vi "sub vi - Read Analog All v8.11.vi"() -> (2 "Analog loop time":dbl, 3 "array GRAPH":dynamicdata[](array[waveform]), 4 "LAB01":T2, 6 "LAB02":T3, 8 "LAB03":T4, 10 "LAB04":T5, 14 "array ERROR":errorcluster[](array[cluster]), 15 "LAB05":T6)   [LabVIEW 2013]
uses:
  program files/Global display 3.vi
  <vilib>/measure/mascope.llb/Amplitude and Levels 1 chan.vi
  <vilib>/addons/Electrical Power/Basic/Measurement/Power (1 Channel).vi
  <vilib>/addons/Electrical Power/Basic/Measurement/RMS (N Channels).vi
  <vilib>/addons/Electrical Power/Basic/NI_EP_Basic.lvlib
  <vilib>/measure/NI_MAPro.lvlib
panel:
  in  "Tab Control":T1(tab)
  out "LAB01-2 (PF)":dbl
  out "LAB01-1 (PF)":dbl
  out "LAB01-2 (V)":dbl
  out "LAB01-2 (A)":dbl
  out "LAB01-1 (V)":dbl
  out "LAB01-1 (A)":dbl
  out "LAB01-2 (GRAPH)":dynamicdata(graph)
  out "LAB01-1 (GRAPH)":dynamicdata(graph)
  out "LAB02-2 (PF)":dbl
  out "LAB02-1 (PF)":dbl
  out "LAB02-2 (V)":dbl
  out "LAB02-2 (A)":dbl
  out "LAB02-1 (V)":dbl
  out "LAB02-1 (A)":dbl
  out "LAB02-2 (GRAPH)":dynamicdata(graph)
  out "LAB02-1 (GRAPH)":dynamicdata(graph)
  out "LAB03-2 (PF)":dbl
  out "LAB03-1 (PF)":dbl
  out "LAB03-2 (V)":dbl
  out "LAB03-2 (A)":dbl
  out "LAB03-1 (V)":dbl
  out "LAB03-1 (A)":dbl
  out "LAB03-2 (GRAPH)":dynamicdata(graph)
  out "LAB03-1 (GRAPH)":dynamicdata(graph)
  out "LAB04-2 (PF)":dbl
  out "LAB04-1 (PF)":dbl
  out "LAB04-2 (V)":dbl
  out "LAB04-2 (A)":dbl
  out "LAB04-1 (V)":dbl
  out "LAB04-1 (A)":dbl
  out "LAB04-1 (GRAPH)":dynamicdata(graph)
  out "LAB04-2 (GRAPH)":dynamicdata(graph)
  out "LAB05-2 (PF)":dbl
  out "LAB05-1 (PF)":dbl
  out "LAB05-2 (V)":dbl
  out "LAB05-2 (A)":dbl
  out "LAB05-1 (V)":dbl
  out "LAB05-1 (A)":dbl
  out "LAB05-1 (GRAPH)":dynamicdata(graph)
  out "LAB05-2 (GRAPH)":dynamicdata(graph)
  out "A1 error":errorcluster
  out "AI2-OFF":dynamicdata(graph)
  out "AI2-ON":dynamicdata(graph)
  out "AI1-OFF":dynamicdata(graph)
  out "AI1-ON":dynamicdata(graph)
  out "AI0-OFF":dynamicdata(graph)
  out "AI0-ON":dynamicdata(graph)
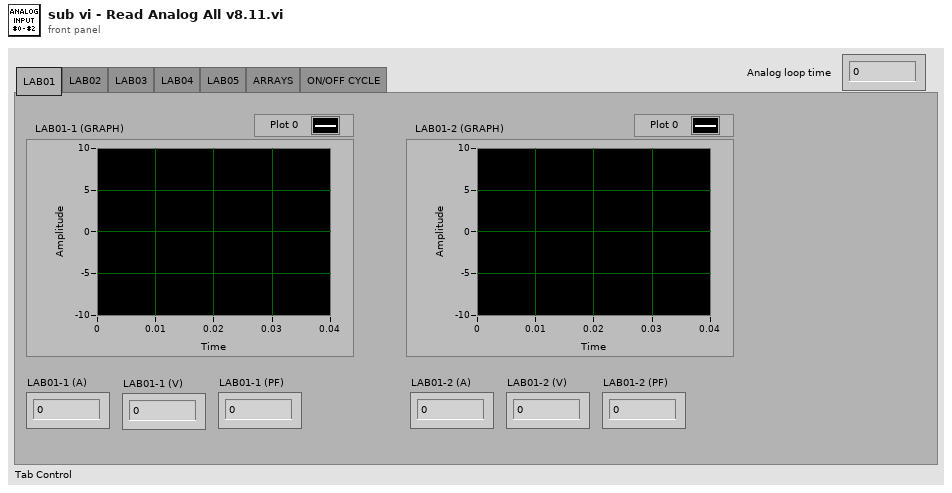
[diagram p1: front panel]
types:
  T1 = enum32{"LAB01", "LAB02", "LAB03", "LAB04", "LAB05", "ARRAYS", "ON/OFF CYCLE"}
  T2 = cluster{"LAB01-1 (A)":dbl, "LAB01-1 (V)":dbl, "LAB01-1 (PF)":dbl, "LAB01-2 (A)":dbl, "LAB01-2 (V)":dbl, "LAB01-2 (PF)":dbl}
  T3 = cluster{"LAB02-1 (A)":dbl, "LAB02-1 (V)":dbl, "LAB02-1 (PF)":dbl, "LAB02-2 (A)":dbl, "LAB02-2 (V)":dbl, "LAB02-2 (PF)":dbl}
  T4 = cluster{"LAB03-1 (A)":dbl, "LAB03-1 (V)":dbl, "LAB03-1 (PF)":dbl, "LAB03-2 (A)":dbl, "LAB03-2 (V)":dbl, "LAB03-2 (PF)":dbl}
  T5 = cluster{"LAB04-1 (A)":dbl, "LAB04-1 (V)":dbl, "LAB04-1 (PF)":dbl, "LAB04-2 (A)":dbl, "LAB04-2 (V)":dbl, "LAB04-2 (PF)":dbl}
  T6 = cluster{"LAB05-1 (A)":dbl, "LAB05-1 (V)":dbl, "LAB05-1 (PF)":dbl, "LAB05-2 (A)":dbl, "LAB05-2 (V)":dbl, "LAB05-2 (PF)":dbl}
  T7 = typedef "NI_EP_Basic.lvlib/basic_Power Value.ctl" = cluster{"active power [W]":dbl, "apparent power [VA]":dbl, "reactive power [VAR]":dbl, "power factor":dbl}
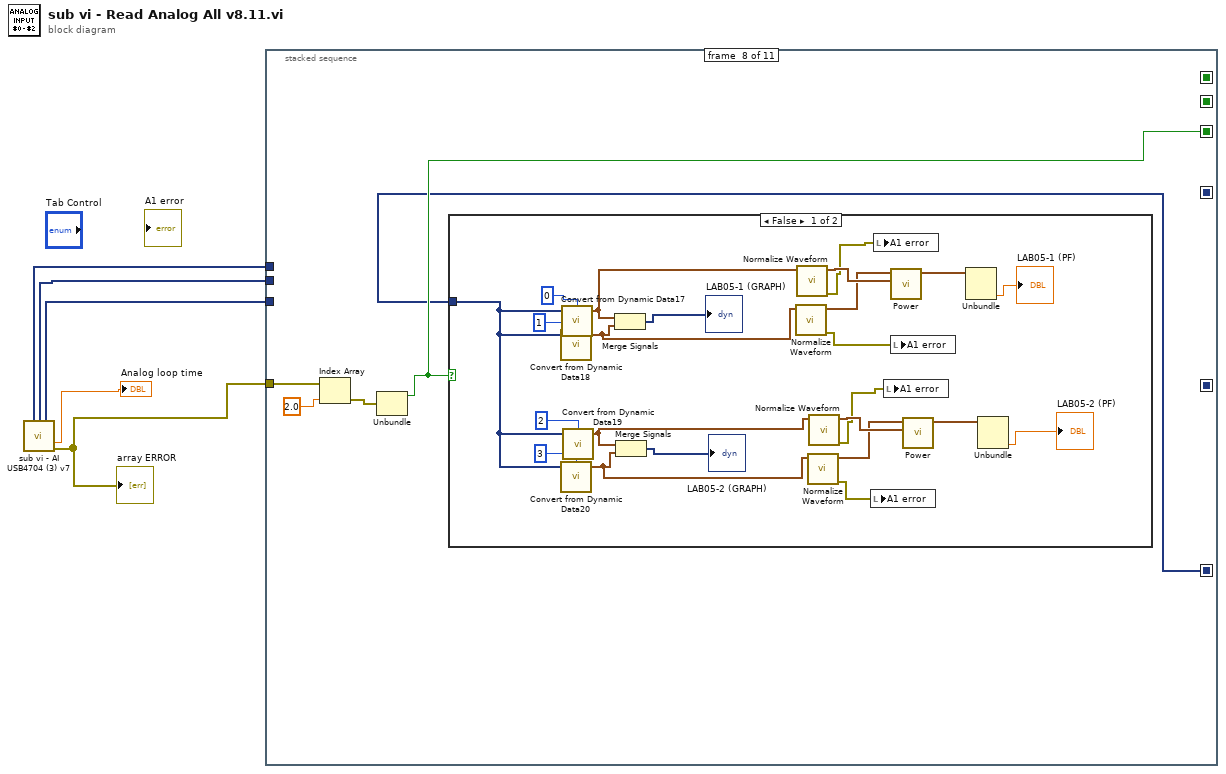
[diagram p0: block diagram]
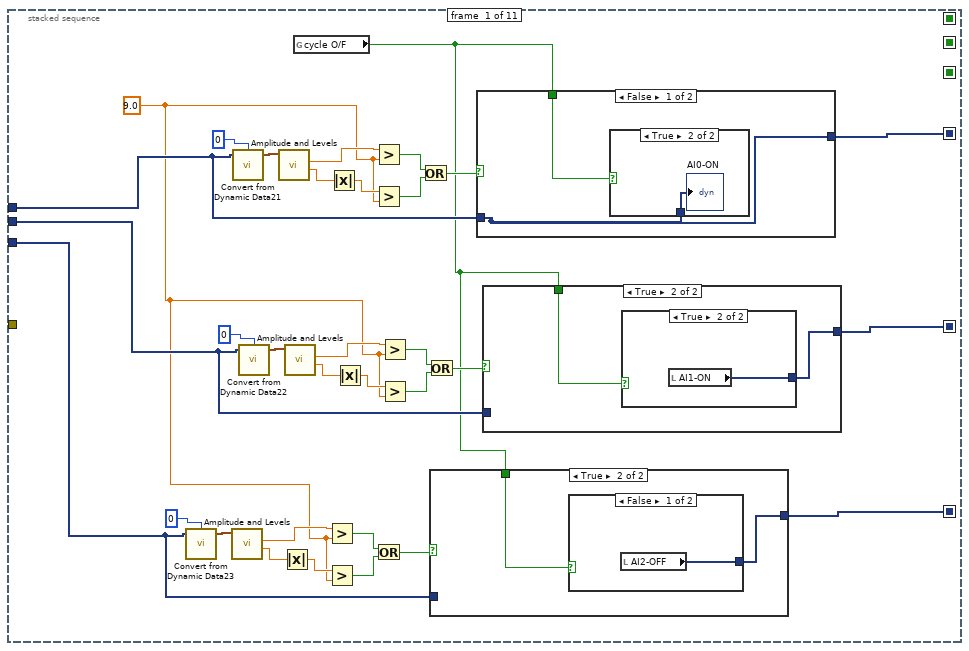
[diagram p2: hidden frame]
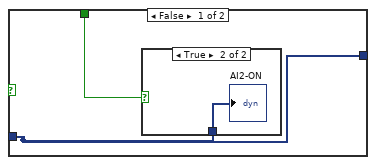
[diagram p3: hidden frame]
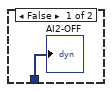
[diagram p4: hidden frame]
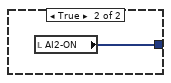
[diagram p5: hidden frame]
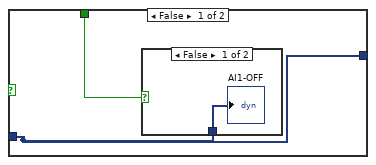
[diagram p6: hidden frame]
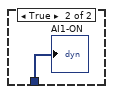
[diagram p7: hidden frame]
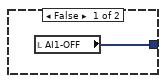
[diagram p8: hidden frame]
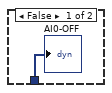
[diagram p9: hidden frame]
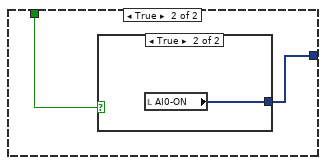
[diagram p10: hidden frame]
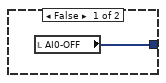
[diagram p11: hidden frame]
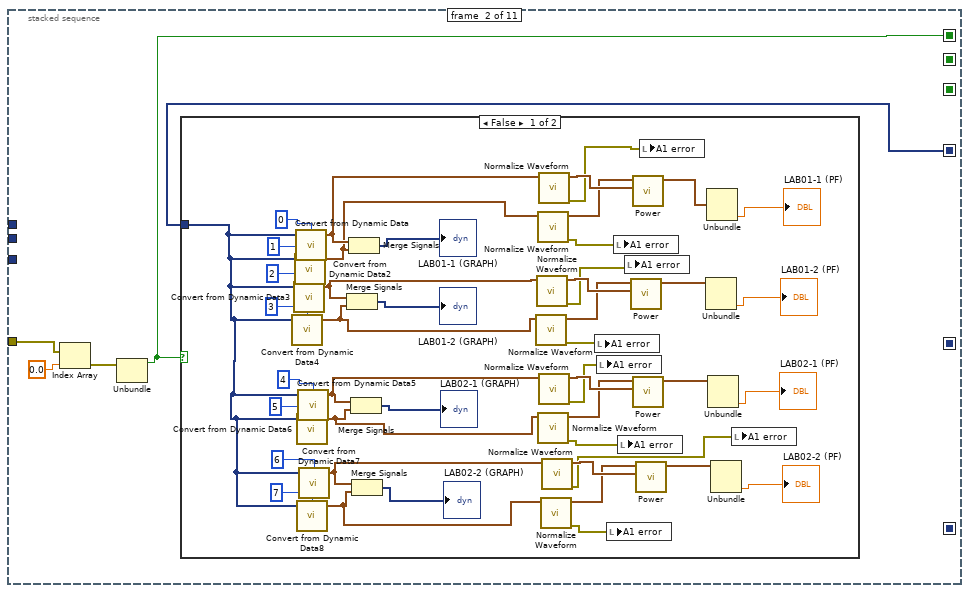
[diagram p12: hidden frame]
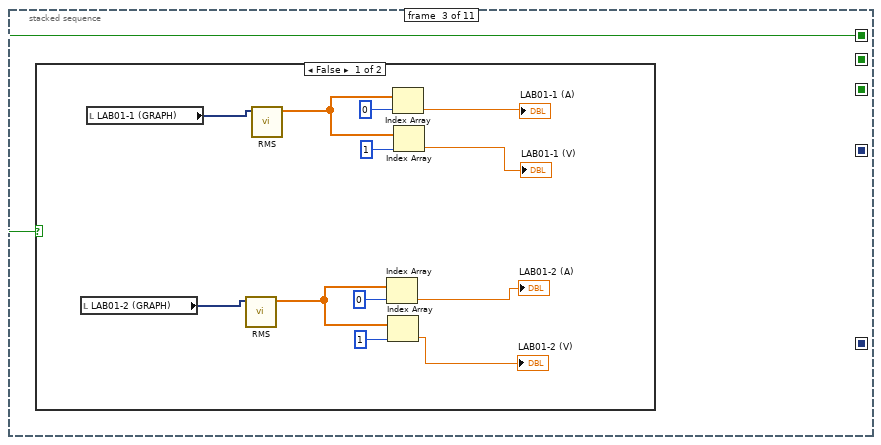
[diagram p14: hidden frame]
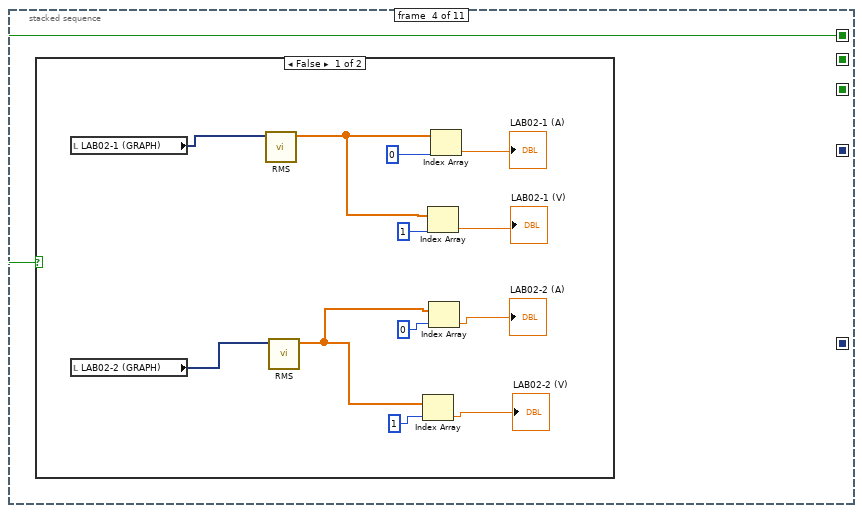
[diagram p16: hidden frame]
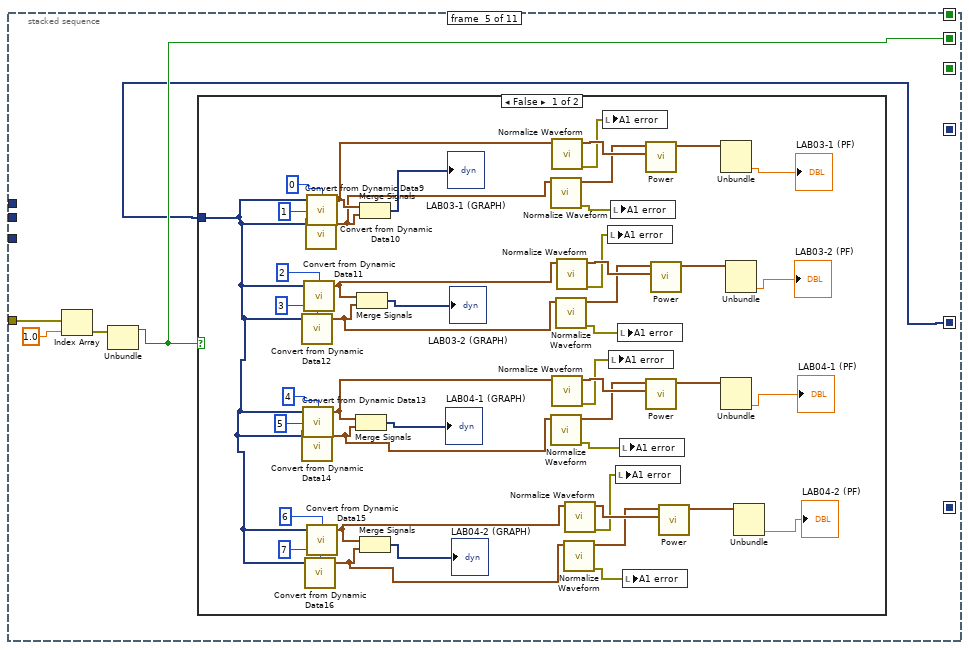
[diagram p18: hidden frame]
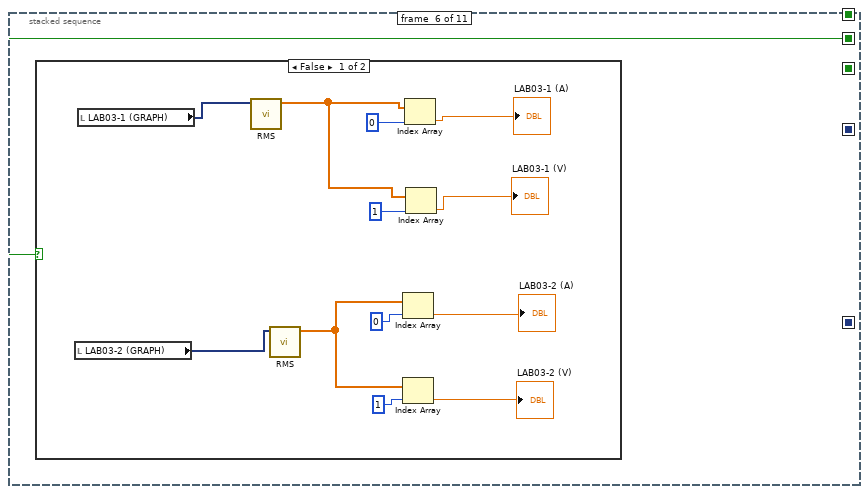
[diagram p20: hidden frame]
diagram:
  n1 = call "sub vi - AI USB4704 (3) v7.vi"() -> ("Graph 1"=w5:dynamicdata, "Graph 2"=w4:dynamicdata, "Graph 3"=w3:dynamicdata, "loop time"=→"Analog loop time":dbl, "error array"=w1:errorcluster[])  [unwired: 11 in]
  "array ERROR" <- w1
  n2 = stacked-sequence {
    seq-local: [_ w63 _ _ _ _ _ _ _ _ _] -> [_ _ w112 w125 _ _ _ _ _ _ w268]
    seq-local: [_ _ _ _ w139 _ _ _ _ _ _] -> [_ _ _ _ _ w188 w201 _ _ _ w267]
    seq-local: [_ _ _ _ _ _ _ w215 _ _ _] -> [_ _ _ _ _ _ _ _ w242 _ w266]
    seq-local: [w29 _ _ _ _ _ _ _ _ _ _] -> [_ w62 _ _ _ _ _ _ _ _ _]
    seq-local: [w18 _ _ _ _ _ _ _ _ _ _] -> [_ _ _ _ w138 _ _ _ _ _ _]
    seq-local: [w6 _ _ _ _ _ _ _ _ _ _] -> [_ _ _ _ _ _ _ w214 _ _ _]
    tunnel: w5 -> [w28 _ _ _ _ _ _ _ _ _ _]
    tunnel: w4 -> [w19 _ _ _ _ _ _ _ _ _ _]
    tunnel: w3 -> [w9 _ _ _ _ _ _ _ _ _ _]
    tunnel: w1 -> [_ w66 _ _ w142 _ _ w218 _ _ _]
    frame #0 {
      w8 = 9.0
      n3 = call "Convert from Dynamic Data23"("Dynamic Data Type"=w9, "Channel"=0) -> ("Waveform"=w16:waveform(dbl))  [unwired: 2 in]
      n4 = call-poly <vilib>:"Amplitude and Levels.vi"("signal in"=w16) -> ("low state level"=w15:dbl, "high state level"=w14:dbl)  [unwired: 7 in, 2 out]
      n5 = call "Convert from Dynamic Data21"("Dynamic Data Type"=w28, "Channel"=0) -> ("Waveform"=w36:waveform(dbl))  [unwired: 2 in]
      n6 = call "Convert from Dynamic Data22"("Dynamic Data Type"=w19, "Channel"=0) -> ("Waveform"=w26:waveform(dbl))  [unwired: 2 in]
      n7 = call-poly <vilib>:"Amplitude and Levels.vi"("signal in"=w36) -> ("low state level"=w35:dbl, "high state level"=w34:dbl)  [unwired: 7 in, 2 out]
      n8 = Absolute Value(x=w15) -> (abs(x)=w13:dbl)
      n9 = call-poly <vilib>:"Amplitude and Levels.vi"("signal in"=w26) -> ("low state level"=w25:dbl, "high state level"=w24:dbl)  [unwired: 7 in, 2 out]
      n10 = global read "Global display 3.vi" "cycle O/F"() -> (w7:bool)
      n11 = Greater?(x=w14, y=w8) -> (0:w12:bool)
      n12 = Greater?(x=w13, y=w8) -> (0:w11:bool)
      n13 = Absolute Value(x=w35) -> (abs(x)=w33:dbl)
      n14 = Absolute Value(x=w25) -> (abs(x)=w23:dbl)
      n15 = Greater?(x=w34, y=w8) -> (0:w32:bool)
      n16 = Greater?(x=w33, y=w8) -> (0:w31:bool)
      n17 = Or(x=w12, y=w11) -> (x .or. y?=w10:bool)
      n18 = Greater?(x=w24, y=w8) -> (0:w22:bool)
      n19 = Greater?(x=w23, y=w8) -> (0:w21:bool)
      n20 = Or(x=w32, y=w31) -> (x .or. y?=w30:bool)
      n21 = Or(x=w22, y=w21) -> (x .or. y?=w20:bool)
      n22 = case shown="True" w10 {
        tunnel: w7 -> [w39 w43]
        tunnel: [w38 w42] -> w6
        tunnel: w9 -> [w38 _]
        frame False {
          n23 = case shown="True" w39 {
            tunnel: w38 -> [w40 w41]
            frame False {
              "AI2-OFF" <- w40
            }
            frame True {
              "AI2-ON" <- w41
            }
          }
        }
        frame True {
          n24 = case shown="False" w43 {
            tunnel: [w44 w45] -> w42
            frame False {
              n25 = local read "AI2-OFF"() -> (w44:dynamicdata)
            }
            frame True {
              n26 = local read "AI2-ON"() -> (w45:dynamicdata)
            }
          }
        }
      }
      n27 = case shown="False" w30 {
        tunnel: w7 -> [w55 w59]
        tunnel: [w54 w58] -> w29
        tunnel: w28 -> [w54 _]
        frame False {
          n28 = case shown="True" w55 {
            tunnel: w54 -> [w56 w57]
            frame False {
              "AI0-OFF" <- w56
            }
            frame True {
              "AI0-ON" <- w57
            }
          }
        }
        frame True {
          n29 = case shown="True" w59 {
            tunnel: [w60 w61] -> w58
            frame False {
              n30 = local read "AI0-OFF"() -> (w60:dynamicdata)
            }
            frame True {
              n31 = local read "AI0-ON"() -> (w61:dynamicdata)
            }
          }
        }
      }
      n32 = case shown="True" w20 {
        tunnel: w7 -> [w47 w51]
        tunnel: [w46 w50] -> w18
        tunnel: w19 -> [w46 _]
        frame False {
          n33 = case shown="False" w47 {
            tunnel: w46 -> [w48 w49]
            frame False {
              "AI1-OFF" <- w48
            }
            frame True {
              "AI1-ON" <- w49
            }
          }
        }
        frame True {
          n34 = case shown="True" w51 {
            tunnel: [w52 w53] -> w50
            frame False {
              n35 = local read "AI1-OFF"() -> (w52:dynamicdata)
            }
            frame True {
              n36 = local read "AI1-ON"() -> (w53:dynamicdata)
            }
          }
        }
      }
    }
    frame #1 {
      n37 = Index Array(array=w66, index=0.0) -> (element=w64:errorcluster)
      n38 = Unbundle(w64) -> ("status"=w63:bool)  [unwired: 2 out]
      n39 = case shown="False" w63 {
        tunnel: w62 -> [w101 _]
        frame False {
          n40 = call "Convert from Dynamic Data4"("Dynamic Data Type"=w101, "Channel"=3) -> ("Waveform"=w87:waveform(dbl))  [unwired: 2 in]
          n41 = call "Convert from Dynamic Data3"("Dynamic Data Type"=w101, "Channel"=2) -> ("Waveform"=w88:waveform(dbl))  [unwired: 2 in]
          n42 = call "Convert from Dynamic Data2"("Dynamic Data Type"=w101, "Channel"=1) -> ("Waveform"=w97:waveform(dbl))  [unwired: 2 in]
          n43 = call "Convert from Dynamic Data"("Dynamic Data Type"=w101, "Channel"=0) -> ("Waveform"=w98:waveform(dbl))  [unwired: 2 in]
          n44 = call "Convert from Dynamic Data6"("Dynamic Data Type"=w101, "Channel"=5) -> ("Waveform"=w82:waveform(dbl))  [unwired: 2 in]
          n45 = call "Convert from Dynamic Data8"("Dynamic Data Type"=w101, "Channel"=7) -> ("Waveform"=w76:waveform(dbl))  [unwired: 2 in]
          n46 = call "Convert from Dynamic Data5"("Dynamic Data Type"=w101, "Channel"=4) -> ("Waveform"=w83:waveform(dbl))  [unwired: 2 in]
          n47 = call "Convert from Dynamic Data7"("Dynamic Data Type"=w101, "Channel"=6) -> ("Waveform"=w77:waveform(dbl))  [unwired: 2 in]
          n48 = Merge Signals(w88, w87) -> (→"LAB01-2 (GRAPH)":dynamicdata)
          n49 = Merge Signals(w98, w97) -> (→"LAB01-1 (GRAPH)":dynamicdata)
          n50 = Merge Signals(w83, w82) -> (→"LAB02-1 (GRAPH)":dynamicdata)
          n51 = Merge Signals(w77, w76) -> (→"LAB02-2 (GRAPH)":dynamicdata)
          n52 = call <vilib>:"Normalize Waveform.vi"("waveform in"=w87) -> ("error out"=w71:errorcluster, "normalized waveform"=w91:waveform(dbl))  [unwired: 7 in, 2 out]
          n53 = call <vilib>:"Normalize Waveform.vi"("waveform in"=w88) -> ("error out"=w72:errorcluster, "normalized waveform"=w92:waveform(dbl))  [unwired: 7 in, 2 out]
          n54 = call <vilib>:"Normalize Waveform.vi"("waveform in"=w97) -> ("error out"=w73:errorcluster, "normalized waveform"=w95:waveform(dbl))  [unwired: 7 in, 2 out]
          n55 = call <vilib>:"Normalize Waveform.vi"("waveform in"=w82) -> ("error out"=w69:errorcluster, "normalized waveform"=w85:waveform(dbl))  [unwired: 7 in, 2 out]
          n56 = call <vilib>:"Normalize Waveform.vi"("waveform in"=w98) -> ("error out"=w74:errorcluster, "normalized waveform"=w96:waveform(dbl))  [unwired: 7 in, 2 out]
          n57 = call <vilib>:"Normalize Waveform.vi"("waveform in"=w83) -> ("error out"=w70:errorcluster, "normalized waveform"=w86:waveform(dbl))  [unwired: 7 in, 2 out]
          n58 = call <vilib>:"Normalize Waveform.vi"("waveform in"=w76) -> ("error out"=w67:errorcluster, "normalized waveform"=w79:waveform(dbl))  [unwired: 7 in, 2 out]
          n59 = call <vilib>:"Normalize Waveform.vi"("waveform in"=w77) -> ("error out"=w68:errorcluster, "normalized waveform"=w80:waveform(dbl))  [unwired: 7 in, 2 out]
          n60 = local write "A1 error"(w71) -> ()
          n61 = local write "A1 error"(w70) -> ()
          n62 = local write "A1 error"(w67) -> ()
          n63 = local write "A1 error"(w73) -> ()
          n64 = local write "A1 error"(w69) -> ()
          n65 = local write "A1 error"(w72) -> ()
          n66 = call-poly <vilib>:"Power.vi"("current waveform"=w92, "voltage waveform"=w91) -> ("power value"=w90:T7)  [unwired: 8 in, 1 out]
          n67 = call-poly <vilib>:"Power.vi"("current waveform"=w96, "voltage waveform"=w95) -> ("power value"=w94:T7)  [unwired: 8 in, 1 out]
          n68 = call-poly <vilib>:"Power.vi"("current waveform"=w86, "voltage waveform"=w85) -> ("power value"=w84:T7)  [unwired: 8 in, 1 out]
          n69 = call-poly <vilib>:"Power.vi"("current waveform"=w80, "voltage waveform"=w79) -> ("power value"=w78:T7)  [unwired: 8 in, 1 out]
          n70 = local write "A1 error"(w74) -> ()
          n71 = Unbundle(w90) -> ("power factor"=→"LAB01-2 (PF)":dbl)  [unwired: 3 out]
          n72 = Unbundle(w94) -> ("power factor"=→"LAB01-1 (PF)":dbl)  [unwired: 3 out]
          n73 = Unbundle(w84) -> ("power factor"=→"LAB02-1 (PF)":dbl)  [unwired: 3 out]
          n74 = Unbundle(w78) -> ("power factor"=→"LAB02-2 (PF)":dbl)  [unwired: 3 out]
          n75 = local write "A1 error"(w68) -> ()
        }
        frame True {
        }
      }
    }
    frame #2 {
      n76 = case shown="False" w112 {
        frame False {
          n77 = local read "LAB01-2 (GRAPH)"() -> (w121:dynamicdata)
          n78 = local read "LAB01-1 (GRAPH)"() -> (w115:dynamicdata)
          n79 = call-poly <vilib>:"RMS.vi"("waveforms"=w121) -> ("RMS values"=w120:dbl[])  [unwired: 9 in, 1 out]
          n80 = call-poly <vilib>:"RMS.vi"("waveforms"=w115) -> ("RMS values"=w124:dbl[])  [unwired: 9 in, 1 out]
          n81 = Index Array(array=w120, index=0) -> (element=→"LAB01-2 (A)":dbl)
          n82 = Index Array(array=w120, index=1) -> (element=→"LAB01-2 (V)":dbl)
          n83 = Index Array(array=w124, index=0) -> (element=→"LAB01-1 (A)":dbl)
          n84 = Index Array(array=w124, index=1) -> (element=→"LAB01-1 (V)":dbl)
        }
        frame True {
        }
      }
    }
    frame #3 {
      n85 = case shown="False" w125 {
        frame False {
          n86 = local read "LAB02-1 (GRAPH)"() -> (w133:dynamicdata)
          n87 = local read "LAB02-2 (GRAPH)"() -> (w129:dynamicdata)
          n88 = call-poly <vilib>:"RMS.vi"("waveforms"=w133) -> ("RMS values"=w132:dbl[])  [unwired: 9 in, 1 out]
          n89 = call-poly <vilib>:"RMS.vi"("waveforms"=w129) -> ("RMS values"=w128:dbl[])  [unwired: 9 in, 1 out]
          n90 = Index Array(array=w128, index=1) -> (element=→"LAB02-2 (V)":dbl)
          n91 = Index Array(array=w132, index=1) -> (element=→"LAB02-1 (V)":dbl)
          n92 = Index Array(array=w128, index=0) -> (element=→"LAB02-2 (A)":dbl)
          n93 = Index Array(array=w132, index=0) -> (element=→"LAB02-1 (A)":dbl)
        }
        frame True {
        }
      }
    }
    frame #4 {
      n94 = Index Array(array=w142, index=1.0) -> (element=w140:errorcluster)
      n95 = Unbundle(w140) -> ("status"=w139:bool)  [unwired: 2 out]
      n96 = case shown="False" w139 {
        tunnel: w138 -> [w175 _]
        frame False {
          n97 = call "Convert from Dynamic Data12"("Dynamic Data Type"=w175, "Channel"=3) -> ("Waveform"=w164:waveform(dbl))  [unwired: 2 in]
          n98 = call "Convert from Dynamic Data14"("Dynamic Data Type"=w175, "Channel"=5) -> ("Waveform"=w158:waveform(dbl))  [unwired: 2 in]
          n99 = call "Convert from Dynamic Data13"("Dynamic Data Type"=w175, "Channel"=4) -> ("Waveform"=w159:waveform(dbl))  [unwired: 2 in]
          n100 = call "Convert from Dynamic Data11"("Dynamic Data Type"=w175, "Channel"=2) -> ("Waveform"=w165:waveform(dbl))  [unwired: 2 in]
          n101 = call "Convert from Dynamic Data16"("Dynamic Data Type"=w175, "Channel"=7) -> ("Waveform"=w152:waveform(dbl))  [unwired: 2 in]
          n102 = call "Convert from Dynamic Data10"("Dynamic Data Type"=w175, "Channel"=1) -> ("Waveform"=w170:waveform(dbl))  [unwired: 2 in]
          n103 = call "Convert from Dynamic Data9"("Dynamic Data Type"=w175, "Channel"=0) -> ("Waveform"=w171:waveform(dbl))  [unwired: 2 in]
          n104 = call "Convert from Dynamic Data15"("Dynamic Data Type"=w175, "Channel"=6) -> ("Waveform"=w153:waveform(dbl))  [unwired: 2 in]
          n105 = Merge Signals(w159, w158) -> (→"LAB04-1 (GRAPH)":dynamicdata)
          n106 = Merge Signals(w165, w164) -> (→"LAB03-2 (GRAPH)":dynamicdata)
          n107 = Merge Signals(w171, w170) -> (→"LAB03-1 (GRAPH)":dynamicdata)
          n108 = Merge Signals(w153, w152) -> (→"LAB04-2 (GRAPH)":dynamicdata)
          n109 = call <vilib>:"Normalize Waveform.vi"("waveform in"=w170) -> ("error out"=w149:errorcluster, "normalized waveform"=w173:waveform(dbl))  [unwired: 7 in, 2 out]
          n110 = call <vilib>:"Normalize Waveform.vi"("waveform in"=w158) -> ("error out"=w145:errorcluster, "normalized waveform"=w161:waveform(dbl))  [unwired: 7 in, 2 out]
          n111 = call <vilib>:"Normalize Waveform.vi"("waveform in"=w171) -> ("error out"=w150:errorcluster, "normalized waveform"=w174:waveform(dbl))  [unwired: 7 in, 2 out]
          n112 = call <vilib>:"Normalize Waveform.vi"("waveform in"=w159) -> ("error out"=w146:errorcluster, "normalized waveform"=w162:waveform(dbl))  [unwired: 7 in, 2 out]
          n113 = call <vilib>:"Normalize Waveform.vi"("waveform in"=w164) -> ("error out"=w147:errorcluster, "normalized waveform"=w167:waveform(dbl))  [unwired: 7 in, 2 out]
          n114 = call <vilib>:"Normalize Waveform.vi"("waveform in"=w165) -> ("error out"=w148:errorcluster, "normalized waveform"=w168:waveform(dbl))  [unwired: 7 in, 2 out]
          n115 = call <vilib>:"Normalize Waveform.vi"("waveform in"=w152) -> ("error out"=w143:errorcluster, "normalized waveform"=w155:waveform(dbl))  [unwired: 7 in, 2 out]
          n116 = call <vilib>:"Normalize Waveform.vi"("waveform in"=w153) -> ("error out"=w144:errorcluster, "normalized waveform"=w156:waveform(dbl))  [unwired: 7 in, 2 out]
          n117 = local write "A1 error"(w150) -> ()
          n118 = local write "A1 error"(w148) -> ()
          n119 = local write "A1 error"(w146) -> ()
          n120 = local write "A1 error"(w149) -> ()
          n121 = local write "A1 error"(w144) -> ()
          n122 = local write "A1 error"(w147) -> ()
          n123 = local write "A1 error"(w145) -> ()
          n124 = local write "A1 error"(w143) -> ()
          n125 = call-poly <vilib>:"Power.vi"("current waveform"=w174, "voltage waveform"=w173) -> ("power value"=w172:T7)  [unwired: 8 in, 1 out]
          n126 = call-poly <vilib>:"Power.vi"("current waveform"=w162, "voltage waveform"=w161) -> ("power value"=w160:T7)  [unwired: 8 in, 1 out]
          n127 = call-poly <vilib>:"Power.vi"("current waveform"=w168, "voltage waveform"=w167) -> ("power value"=w166:T7)  [unwired: 8 in, 1 out]
          n128 = call-poly <vilib>:"Power.vi"("current waveform"=w156, "voltage waveform"=w155) -> ("power value"=w154:T7)  [unwired: 8 in, 1 out]
          n129 = Unbundle(w172) -> ("power factor"=→"LAB03-1 (PF)":dbl)  [unwired: 3 out]
          n130 = Unbundle(w160) -> ("power factor"=→"LAB04-1 (PF)":dbl)  [unwired: 3 out]
          n131 = Unbundle(w166) -> ("power factor"=→"LAB03-2 (PF)":dbl)  [unwired: 3 out]
          n132 = Unbundle(w154) -> ("power factor"=→"LAB04-2 (PF)":dbl)  [unwired: 3 out]
        }
        frame True {
        }
      }
    }
    frame #5 {
      n133 = case shown="False" w188 {
        frame False {
          n134 = local read "LAB03-2 (GRAPH)"() -> (w195:dynamicdata)
          n135 = local read "LAB03-1 (GRAPH)"() -> (w196:dynamicdata)
          n136 = call-poly <vilib>:"RMS.vi"("waveforms"=w196) -> ("RMS values"=w194:dbl[])  [unwired: 9 in, 1 out]
          n137 = call-poly <vilib>:"RMS.vi"("waveforms"=w195) -> ("RMS values"=w191:dbl[])  [unwired: 9 in, 1 out]
          n138 = Index Array(array=w191, index=0) -> (element=→"LAB03-2 (A)":dbl)
          n139 = Index Array(array=w191, index=1) -> (element=→"LAB03-2 (V)":dbl)
          n140 = Index Array(array=w194, index=0) -> (element=→"LAB03-1 (A)":dbl)
          n141 = Index Array(array=w194, index=1) -> (element=→"LAB03-1 (V)":dbl)
        }
        frame True {
        }
      }
    }
    frame #6 {
      n142 = case shown="False" w201 {
        frame False {
          n143 = local read "LAB04-1 (GRAPH)"() -> (w209:dynamicdata)
          n144 = local read "LAB04-2 (GRAPH)"() -> (w205:dynamicdata)
          n145 = call-poly <vilib>:"RMS.vi"("waveforms"=w209) -> ("RMS values"=w208:dbl[])  [unwired: 9 in, 1 out]
          n146 = call-poly <vilib>:"RMS.vi"("waveforms"=w205) -> ("RMS values"=w204:dbl[])  [unwired: 9 in, 1 out]
          n147 = Index Array(array=w204, index=0) -> (element=→"LAB04-2 (A)":dbl)
          n148 = Index Array(array=w208, index=0) -> (element=→"LAB04-1 (A)":dbl)
          n149 = Index Array(array=w204, index=1) -> (element=→"LAB04-2 (V)":dbl)
          n150 = Index Array(array=w208, index=1) -> (element=→"LAB04-1 (V)":dbl)
        }
        frame True {
        }
      }
    }
    frame #7 {
      n151 = Index Array(array=w218, index=2.0) -> (element=w216:errorcluster)
      n152 = Unbundle(w216) -> ("status"=w215:bool)  [unwired: 2 out]
      n153 = case shown="False" w215 {
        tunnel: w214 -> [w235 _]
        frame False {
          n154 = call "Convert from Dynamic Data18"("Dynamic Data Type"=w235, "Channel"=1) -> ("Waveform"=w230:waveform(dbl))  [unwired: 2 in]
          n155 = call "Convert from Dynamic Data20"("Dynamic Data Type"=w235, "Channel"=3) -> ("Waveform"=w224:waveform(dbl))  [unwired: 2 in]
          n156 = call "Convert from Dynamic Data17"("Dynamic Data Type"=w235, "Channel"=0) -> ("Waveform"=w231:waveform(dbl))  [unwired: 2 in]
          n157 = call "Convert from Dynamic Data19"("Dynamic Data Type"=w235, "Channel"=2) -> ("Waveform"=w225:waveform(dbl))  [unwired: 2 in]
          n158 = Merge Signals(w231, w230) -> (→"LAB05-1 (GRAPH)":dynamicdata)
          n159 = Merge Signals(w225, w224) -> (→"LAB05-2 (GRAPH)":dynamicdata)
          n160 = call <vilib>:"Normalize Waveform.vi"("waveform in"=w230) -> ("error out"=w222:errorcluster, "normalized waveform"=w233:waveform(dbl))  [unwired: 7 in, 2 out]
          n161 = call <vilib>:"Normalize Waveform.vi"("waveform in"=w231) -> ("error out"=w221:errorcluster, "normalized waveform"=w234:waveform(dbl))  [unwired: 7 in, 2 out]
          n162 = call <vilib>:"Normalize Waveform.vi"("waveform in"=w224) -> ("error out"=w220:errorcluster, "normalized waveform"=w227:waveform(dbl))  [unwired: 7 in, 2 out]
          n163 = call <vilib>:"Normalize Waveform.vi"("waveform in"=w225) -> ("error out"=w219:errorcluster, "normalized waveform"=w228:waveform(dbl))  [unwired: 7 in, 2 out]
          n164 = local write "A1 error"(w220) -> ()
          n165 = local write "A1 error"(w221) -> ()
          n166 = local write "A1 error"(w219) -> ()
          n167 = call-poly <vilib>:"Power.vi"("current waveform"=w234, "voltage waveform"=w233) -> ("power value"=w232:T7)  [unwired: 8 in, 1 out]
          n168 = local write "A1 error"(w222) -> ()
          n169 = call-poly <vilib>:"Power.vi"("current waveform"=w228, "voltage waveform"=w227) -> ("power value"=w226:T7)  [unwired: 8 in, 1 out]
          n170 = Unbundle(w232) -> ("power factor"=→"LAB05-1 (PF)":dbl)  [unwired: 3 out]
          n171 = Unbundle(w226) -> ("power factor"=→"LAB05-2 (PF)":dbl)  [unwired: 3 out]
        }
        frame True {
        }
      }
    }
    frame #8 {
      n172 = case shown="False" w242 {
        frame False {
          n173 = local read "LAB05-2 (GRAPH)"() -> (w249:dynamicdata)
          n174 = local read "LAB05-1 (GRAPH)"() -> (w250:dynamicdata)
          n175 = call-poly <vilib>:"RMS.vi"("waveforms"=w250) -> ("RMS values"=w248:dbl[])  [unwired: 9 in, 1 out]
          n176 = call-poly <vilib>:"RMS.vi"("waveforms"=w249) -> ("RMS values"=w247:dbl[])  [unwired: 9 in, 1 out]
          n177 = Index Array(array=w248, index=1) -> (element=→"LAB05-1 (V)":dbl)
          n178 = Index Array(array=w248, index=0) -> (element=→"LAB05-1 (A)":dbl)
          n179 = Index Array(array=w247, index=1) -> (element=→"LAB05-2 (V)":dbl)
          n180 = Index Array(array=w247, index=0) -> (element=→"LAB05-2 (A)":dbl)
        }
        frame True {
        }
      }
    }
    frame #9 {
      n181 = local read "LAB05-1 (GRAPH)"() -> (w257:dynamicdata)
      n182 = local read "LAB05-2 (GRAPH)"() -> (w256:dynamicdata)
      n183 = local read "LAB04-2 (GRAPH)"() -> (w258:dynamicdata)
      n184 = local read "LAB02-2 (GRAPH)"() -> (w262:dynamicdata)
      n185 = local read "LAB03-1 (GRAPH)"() -> (w261:dynamicdata)
      n186 = local read "LAB04-1 (GRAPH)"() -> (w259:dynamicdata)
      n187 = local read "LAB03-2 (GRAPH)"() -> (w260:dynamicdata)
      n188 = local read "LAB02-1 (GRAPH)"() -> (w263:dynamicdata)
      n189 = local read "LAB01-2 (GRAPH)"() -> (w264:dynamicdata)
      n190 = local read "LAB01-1 (GRAPH)"() -> (w265:dynamicdata)
      n191 = Build Array(w265, w264, w263, w262, w261, w260, w259, w258, w257, w256) -> (→"array GRAPH":dynamicdata[])
    }
    frame #10 {
      n192 = case shown="False" w267 {
        frame False {
          n193 = local read "LAB03-2 (PF)"() -> (w284:dbl)
          n194 = local read "LAB03-1 (PF)"() -> (w287:dbl)
          n195 = local read "LAB03-1 (A)"() -> (w289:dbl)
          n196 = local read "LAB03-1 (V)"() -> (w288:dbl)
          n197 = local read "LAB03-2 (A)"() -> (w286:dbl)
          n198 = local read "LAB03-2 (V)"() -> (w285:dbl)
          n199 = Bundle("LAB03-1 (A)"=w289, "LAB03-1 (V)"=w288, "LAB03-1 (PF)"=w287, "LAB03-2 (A)"=w286, "LAB03-2 (V)"=w285, "LAB03-2 (PF)"=w284) -> (→"LAB03":T4)  [unwired: 1 in]
          n200 = local read "LAB04-1 (PF)"() -> (w281:dbl)
          n201 = local read "LAB04-2 (PF)"() -> (w278:dbl)
          n202 = local read "LAB04-1 (A)"() -> (w283:dbl)
          n203 = local read "LAB04-1 (V)"() -> (w282:dbl)
          n204 = local read "LAB04-2 (A)"() -> (w280:dbl)
          n205 = local read "LAB04-2 (V)"() -> (w279:dbl)
          n206 = Bundle("LAB04-1 (A)"=w283, "LAB04-1 (V)"=w282, "LAB04-1 (PF)"=w281, "LAB04-2 (A)"=w280, "LAB04-2 (V)"=w279, "LAB04-2 (PF)"=w278) -> (→"LAB04":T5)  [unwired: 1 in]
        }
        frame True {
        }
      }
      n207 = case shown="False" w268 {
        frame False {
          n208 = local read "LAB01-1 (PF)"() -> (w294:dbl)
          n209 = local read "LAB01-2 (PF)"() -> (w291:dbl)
          n210 = local read "LAB01-1 (V)"() -> (w295:dbl)
          n211 = local read "LAB01-2 (A)"() -> (w293:dbl)
          n212 = local read "LAB01-2 (V)"() -> (w292:dbl)
          n213 = local read "LAB01-1 (A)"() -> (w296:dbl)
          n214 = Bundle("LAB01-1 (A)"=w296, "LAB01-1 (V)"=w295, "LAB01-1 (PF)"=w294, "LAB01-2 (A)"=w293, "LAB01-2 (V)"=w292, "LAB01-2 (PF)"=w291) -> (→"LAB01":T2)  [unwired: 1 in]
          n215 = local read "LAB02-2 (PF)"() -> (w298:dbl)
          n216 = local read "LAB02-1 (PF)"() -> (w301:dbl)
          n217 = local read "LAB02-2 (A)"() -> (w300:dbl)
          n218 = local read "LAB02-2 (V)"() -> (w299:dbl)
          n219 = local read "LAB02-1 (V)"() -> (w302:dbl)
          n220 = local read "LAB02-1 (A)"() -> (w303:dbl)
          n221 = Bundle("LAB02-1 (A)"=w303, "LAB02-1 (V)"=w302, "LAB02-1 (PF)"=w301, "LAB02-2 (A)"=w300, "LAB02-2 (V)"=w299, "LAB02-2 (PF)"=w298) -> (→"LAB02":T3)  [unwired: 1 in]
        }
        frame True {
        }
      }
      n222 = case shown="False" w266 {
        frame False {
          n223 = local read "LAB05-2 (PF)"() -> (w270:dbl)
          n224 = local read "LAB05-1 (PF)"() -> (w273:dbl)
          n225 = local read "LAB05-2 (V)"() -> (w271:dbl)
          n226 = local read "LAB05-1 (A)"() -> (w275:dbl)
          n227 = local read "LAB05-1 (V)"() -> (w274:dbl)
          n228 = local read "LAB05-2 (A)"() -> (w272:dbl)
          n229 = Bundle("LAB05-1 (A)"=w275, "LAB05-1 (V)"=w274, "LAB05-1 (PF)"=w273, "LAB05-2 (A)"=w272, "LAB05-2 (V)"=w271, "LAB05-2 (PF)"=w270) -> (→"LAB05":T6)  [unwired: 1 in]
        }
        frame True {
        }
      }
    }
  }
